vi "CCD Acquire Spectrum and Abort Acquisition.vi"(11 "error in":errorcluster) -> (15 "error out":errorcluster)   [LabVIEW 2020, in "Examples.lvlib"]
doc: "Example for a CCD spectrum acquisition."
uses:
  Examples.lvlib
  Classes/CCD/TriggerIn.ctl
  4aef6941-9f58-45d1-a797-2b486d7897ac.vi
  5e6a2402-05de-4989-a080-2a16ebe75cc4.vi
  Classes/CCD/CCD.lvclass
panel:
  out "isBusy after Abort":bool
  out "isBusy before Abort":bool
  # "Connector Pane"
  # "Locals"
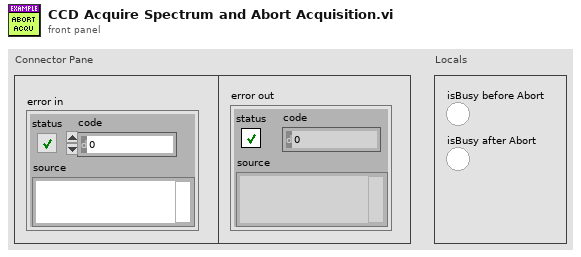
[diagram p1: front panel]
types:
  T1 = typedef "horiba.lvlib/CCD.lvclass/TriggerIn.ctl" = cluster{"address":i32, "event":i32, "signalType":i32}
  T2 = cluster{"ROI-index":i32, "xOrigin":i32, "yOrigin":i32, "xSize":i32, "ySize":i32, "xBin":i32, "yBin":i32}
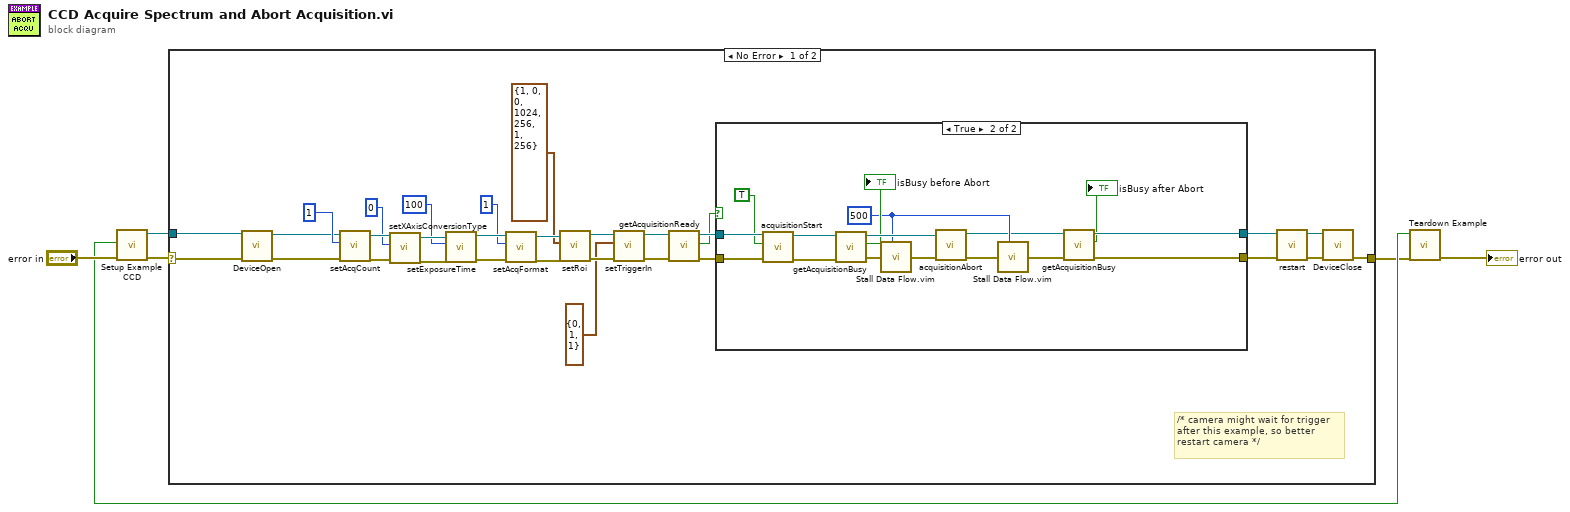
[diagram p0: block diagram]
diagram:
  n1 = call "Setup Example CCD.vi"("error in (no error)"="error in") -> ("error out"=w4:errorcluster, "Module Was Already Running?"=w2:bool, "CCD out"=w3:refnum<class "CCD.lvclass">)  [unwired: 8 in]
  n2 = case shown="No Error" w4 {
    selector: w4 -> [w36 w55]
    tunnel: w3 -> [w15 _]
    tunnel: [w18 w55] -> w1
    frame No Error {
      # "/* camera might wait for trigger\nafter this example, so better \nrestart camera */"
      n3 = call-dynamic "DeviceOpen.vi"("error in (no error)"=w36, "CCD in"=w15) -> ("error out"=w16:errorcluster, "CCD out"=w14:refnum<class "CCD.lvclass">)  [unwired: 6 in, 2 out]
      n4 = call "setAcqCount.vi"("error in (no error)"=w16, "count"=1, "CCD in"=w14) -> ("error out"=w34:errorcluster, "CCD out"=w33:refnum<class "CCD.lvclass">)  [unwired: 5 in, 2 out]
      n5 = call "setXAxisConversionType.vi"("error in (no error)"=w34, "type"=0, "CCD in"=w33) -> ("error out"=w31:errorcluster, "CCD out"=w30:refnum<class "CCD.lvclass">)  [unwired: 5 in, 2 out]
      n6 = call "setExposureTime.vi"("error in (no error)"=w31, "exposure time [ms] or [us]"=100, "CCD in"=w30) -> ("error out"=w28:errorcluster, "CCD out"=w27:refnum<class "CCD.lvclass">)  [unwired: 5 in, 2 out]
      n7 = call "setAcqFormat.vi"("error in (no error)"=w28, "number of ROIs"=1, "CCD in"=w27) -> ("error out"=w25:errorcluster, "CCD out"=w24:refnum<class "CCD.lvclass">)  [unwired: 5 in, 2 out]
      n8 = call "setRoi.vi"("error in (no error)"=w25, "roiConfig"=T2 {"ROI-index"=1, "xOrigin"=0, "yOrigin"=0, "xSize"=1024, "ySize"=256, "xBin"=1, "yBin"=256}, "CCD in"=w24) -> ("error out"=w23:errorcluster, "CCD out"=w12:refnum<class "CCD.lvclass">)  [unwired: 5 in, 2 out]
      n9 = call "setTriggerIn.vi"("error in (no error)"=w23, "Trigger IN"=T1 {"address"=0, "event"=1, "signalType"=1}, "CCD in"=w12) -> ("error out"=w13:errorcluster, "CCD out"=w11:refnum<class "CCD.lvclass">)  [unwired: 5 in, 2 out]
      n10 = call "getAcquisitionReady.vi"("error in (no error)"=w13, "CCD in"=w11) -> ("error out"=w22:errorcluster, "ready"=w20:bool, "CCD out"=w21:refnum<class "CCD.lvclass">)  [unwired: 7 in]
      n11 = case shown="True" w20 {
        tunnel: w22 -> [w37 w54]
        tunnel: w21 -> [w38 w53]
        tunnel: [w37 w42] -> w19
        tunnel: [w38 w40] -> w8
        frame False {
        }
        frame True {
          w43 = u32 500 ("milliseconds to wait")
          n12 = call "acquisitionStart.vi"("error in (no error)"=w54, "openShutter"=TRUE, "CCD in"=w53) -> ("error out"=w50:errorcluster, "CCD out"=w49:refnum<class "CCD.lvclass">)  [unwired: 5 in, 2 out]
          n13 = call "getAcquisitionBusy.vi"("error in (no error)"=w50, "CCD in"=w49) -> ("error out"=w46:errorcluster, "isBusy"=→"isBusy before Abort":bool, "CCD out"=w47:refnum<class "CCD.lvclass">)  [unwired: 7 in]
          n14 = call "Stall Data Flow.vim"("value in"=w46, "milliseconds to wait"=w43) -> ("value out"=w51:errorcluster)  [unwired: 1 out]
          n15 = call "acquisitionAbort.vi"("error in (no error)"=w51, "CCD in"=w47) -> ("error out"=w48:errorcluster, "CCD out"=w41:refnum<class "CCD.lvclass">)  [unwired: 6 in, 2 out]
          n16 = call "Stall Data Flow.vim"("value in"=w48, "milliseconds to wait"=w43) -> ("value out"=w44:errorcluster)  [unwired: 1 out]
          n17 = call "getAcquisitionBusy.vi"("error in (no error)"=w44, "CCD in"=w41) -> ("error out"=w42:errorcluster, "isBusy"=→"isBusy after Abort":bool, "CCD out"=w40:refnum<class "CCD.lvclass">)  [unwired: 7 in]
        }
      }
      n18 = call "restart.vi"("error in (no error)"=w19, "CCD in"=w8) -> ("error out"=w9:errorcluster, "CCD out"=w7:refnum<class "CCD.lvclass">)  [unwired: 6 in, 2 out]
      n19 = call-dynamic "DeviceClose.vi"("error in (no error)"=w9, "CCD in"=w7) -> ("error out"=w18:errorcluster)  [unwired: 5 in, 4 out]
    }
    frame Error {
    }
  }
  n20 = call "Teardown Example.vi"("error in (no error)"=w1, "Module Was Already Running?"=w2) -> ("error out"=→"error out":errorcluster)  [unwired: 9 in]
